vi "Read Project Reference.vi"(8 "error in (no error)":errorcluster, 11 "LabVIEW Build Script in":refnum<class "LabVIEW Build Script.lvclass">) -> (0 "error out":errorcluster, 2 "Project Reference":refnum<vi>, 3 "LabVIEW Build Script out":refnum<class "LabVIEW Build Script.lvclass">)   [LabVIEW 2021, in "LabVIEW Build Script.lvclass"]
uses:
  LabVIEW Build Script.lvclass
  LabVIEW Build Script.lvclass/LabVIEW Build Script.ctl
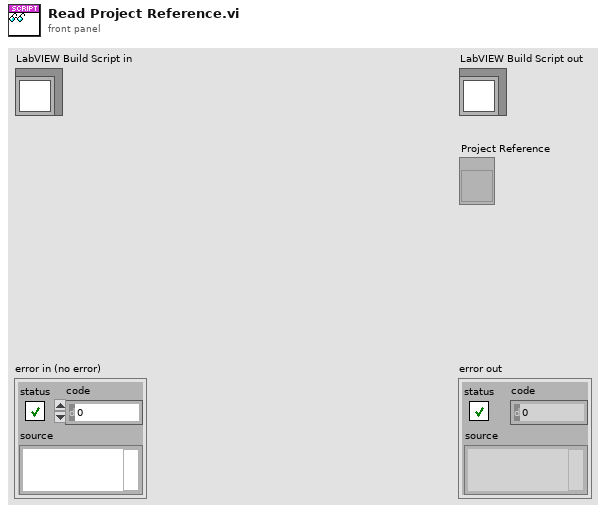
[diagram p1: front panel]
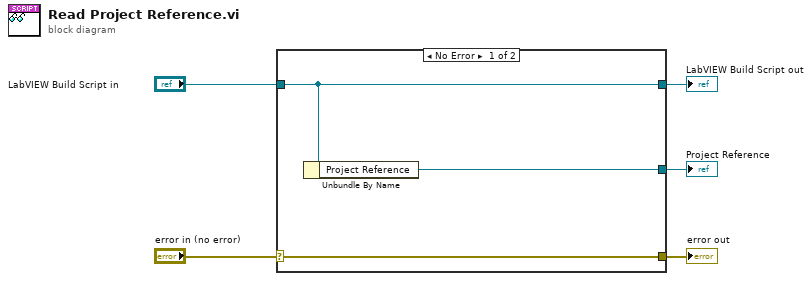
[diagram p0: block diagram]
diagram:
  n1 = case shown="No Error" "error in (no error)" {
    selector: "error in (no error)" -> [w8 w9]
    tunnel: [w8 w9] -> w4
    tunnel: [w7 w10] -> w2
    tunnel: "LabVIEW Build Script in" -> [w7 w10]
    tunnel: [w6 _] -> w1
    frame No Error {
      n2 = Unbundle By Name(w7) -> ("Project Reference"=w6:refnum<vi>)
    }
    frame Error {
    }
  }
  "error out" <- w4
  "LabVIEW Build Script out" <- w2
  "Project Reference" <- w1
